vi "Get_USER_ID.vi"(8 "错误输入":errorcluster, 11 "USER_EMPLOYEE_ID":string) -> (0 "错误输出":errorcluster, 3 "USER_ID":string)   [LabVIEW 2020]
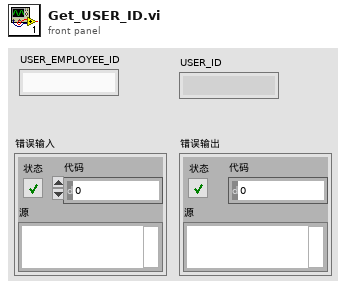
[diagram p1: front panel]
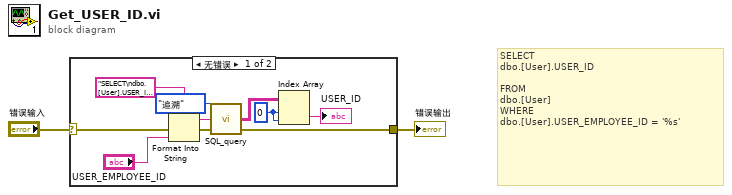
[diagram p0: block diagram]
diagram:
  # "SELECT\ndbo.[User].USER_ID\n\nFROM\ndbo.[User]\nWHERE\ndbo.[User].USER_EMPLOYEE_ID = '%s'"
  n1 = case shown="无错误" "错误输入" {
    selector: "错误输入" -> [w9 w13]
    tunnel: [w7 w13] -> w1
    frame No Error {
      w11 = 0 ("索引 (行)")
      n2 = Format Into String(format string="SELECT\ndbo.[User].USER_ID\n\nFROM\ndbo.[User]\nWHERE\ndbo.[User].USER_EMPLOYEE_ID = '%s'\n", error in=w9, "USER_EMPLOYEE_ID") -> (resulting string=w12:string, error out=w8:errorcluster)  [unwired: 1 in]
      n3 = call "SQL_query.vi"("error in (no error)"=w8, "SQL query"=w12, "联机模式"=enum16{"单机", "追溯"}."追溯") -> ("error out"=w7:errorcluster, "data"=w6:string[][])  [unwired: 1 out]
      n4 = Index Array(array=w6, index (row)=w11, index (col)=w11) -> (element=→"USER_ID":string)
    }
    frame Error {
    }
  }
  "错误输出" <- w1
